vi "Main.vi"() -> ()   [LabVIEW 2021]
uses:
  <vilib>/rvi/DesktopExecutionNode/Execution/niFpgaDEN_Execute.vi
  <vilib>/rvi/DesktopExecutionNode/DesktopExecutionNode.xnode
panel:
  out "LED3":bool
  out "LED0":bool
  out "Button 0":bool
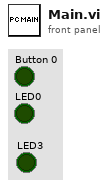
[diagram p1: front panel]
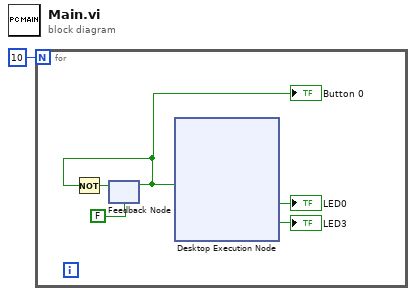
[diagram p0: block diagram]
diagram:
  n1 = for {
    N: 10 -> [_]
    n2 = feedback #1(FALSE) -> (w4:bool)
    "Button 0" <- w4
    n3 = Not(x=w4) -> (.not. x?=w5:bool)
    n4 = feedback-in #1(w5) -> ()
    n5 = xnode "Desktop Execution Node"("Button0"=w4) -> ("LED0"=→"LED0":bool, "LED3"=→"LED3":bool)  [unwired: 1 in, 1 out]
  }
